vi "Begin.vi"(8 "error in":errorcluster) -> (0 "error out":errorcluster)   [LabVIEW 2014]
doc: "Called before other user functions, this VI is expected to open initial I/O refnums, load in file data, and do all program initialization. Notice that the <B>error out</B> terminal is simply used for data flow. Wiring it to other structures or subVIs ensures that this VI runs first."
uses:
  <vilib>/Rock Robotics/WPI/SafetyOutput/WPI_SafetyOutputConfigMenu.ctl
  <vilib>/Rock Robotics/WPI/DriverStation/WPI_DriverStationRobotMode2.ctl
  <vilib>/Rock Robotics/SystemInterfaces/AI/FPGA_AIGyroChannel.ctl
  <vilib>/Rock Robotics/SystemInterfaces/AI/FPGA_AIChannel.ctl
  Utilities/Sensor Refname.ctl
  <vilib>/Rock Robotics/SystemInterfaces/DIO/FPGA_DIOChannel.ctl
  Utilities/Refname.ctl
  <vilib>/Rock Robotics/WPI/Joystick/WPI_JoystickDeviceEnum.ctl
  <vilib>/Rock Robotics/WPI/CAN/TalonSRX/WPI_CANTalonSRX_APIControlMode.ctl
  <vilib>/Rock Robotics/WPI/CAN/TalonSRX/WPI_CANTalonSRX_APIFeedbackSelect.ctl
  Robot Global Data.vi
  <vilib>/Rock Robotics/WPI/RobotDrive/WPI_RobotDriveOpen4MotorWithCANTalonSRX.vi
  <vilib>/Rock Robotics/Network Tables/SD Write String.vi
  <vilib>/Rock Robotics/WPI/Switch/WPI_SwitchOpenLimit.vi
  Utilities/Sensor Refname to String.vi
  Utilities/RefnameToString.vi
  <vilib>/Rock Robotics/WPI/Ultrasonic/WPI_SonarMB1010AnalogOpen.vi
  <vilib>/Rock Robotics/WPI/Ultrasonic/WPI_SonarMB1010AnalogRefNum Registry Set.vi
  <vilib>/Rock Robotics/WPI/MotorControl/WPI_MotorControlOpenCANTalonSRX.vi
  <vilib>/Rock Robotics/WPI/Accelerometer/InternalAccelerometer/WPI_AccelerometerInternalOpen.vi
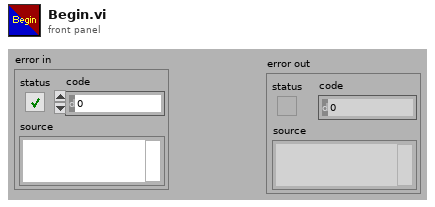
[diagram p1: front panel]
types:
  T1 = typedef "Refname.ctl" = enum16{"Gamepad 1", "Gamepad 2", "Drive Motors", "Strafe Motor", "Arm Clapper Motor", "Arm Angle", "Arm Belt Left", "Arm Belt Right", "Elevator 1", "Elevator 2", "Wiper"}
  T2 = cluster{"Refname":T1, "Device":u8, "Invert?":bool}[]
  T3 = typedef "WPI_JoystickDeviceEnum.ctl" = enum16{"USB 0", "USB 1", "USB 2", "USB 3", "USB 4", "USB 5"}
  T4 = typedef "Sensor Refname.ctl" = enum16{"Gyro", "Elevator Top LS", "Elevator Bottom LS", "Claw Outside LS", "Left Drive Encoder", "Right Drive Encoder", "Strafe Encoder", "Elevator Encoder", "Ultrasonic Forward", "Ultrasonic Back", "Arm Angle POT", "Arm Clapper POT", "Accelerometer", "Tote LS", "DIP 1", "DIP 2", "DIP 3", "DIP 4"}
  T5 = typedef "FPGA_AIChannel.ctl" = enum8{"AI 0", "AI 1", "AI 2", "AI 3", "AI MXP 0", "AI MXP 1", "AI MXP 2", "AI MXP 3", "Invalid"}
  T6 = cluster{"Sensor Refname":T4, "Analog Channel":T5}[]
  T7 = typedef "FPGA_DIOChannel.ctl" = enum8{"DIO 0", "DIO 1", "DIO 2", "DIO 3", "DIO 4", "DIO 5", "DIO 6", "DIO 7", "DIO 8", "DIO 9", "DIO MXP 0", "DIO MXP 1", "DIO MXP 2", "DIO MXP 3", "DIO MXP 4", "DIO MXP 5", "DIO MXP 6", "DIO MXP 7", "DIO MXP 8", "DIO MXP 9", "DIO MXP 10", "DIO MXP 11", "DIO MXP 12", "DIO MXP 13", "DIO MXP 14", "DIO MXP 15", "Invalid"}
  T8 = typedef "FPGA_AIGyroChannel.ctl" = enum8{"AI 0", "AI 1", "Invalid"}
  T9 = typedef "WPI_DriverStationRobotMode2.ctl" = enum16{"Autonomous Disabled", "Autonomous Enabled", "Teleop Disabled", "Teleop Enabled", "Disconnected", "Finish", "Test Disabled", "Test Enabled", "Emergency Stopped"}
  T10 = typedef "WPI_SafetyOutputConfigMenu.ctl" = enum16{"Enable", "Disable"}
  T11 = typedef "WPI_RobotDriveDevRef.ctl" = cluster{"DevStatus":errorcluster, "Motors[]":T12[], "Square Inputs":bool, "Max Output":dbl}
  T12 = typedef "WPI_MotorControlDeviceRef.ctl" = cluster{"DeviceStatus":errorcluster, "Type":T13, "PWM":cluster{"Controller":T14, "PWM Channel":T15, "DeadBand":T16}, "CAN":cluster{"Device Number":u8, "Control Mode":T17, "Semaphore":T18, "Max Vout":dbl, "TalonSRX Control Mode":T19}, "Invert":bool, "TransformRef":T20, "InvTransformRef":T20}
  T13 = typedef "WPI_MotorControlType.ctl" = enum16{"PWM", "CAN", "CANTalonSRX"}
  T14 = typedef "FPGA_TypedefDigitalModule.ctl" = enum16{"Controller 1"}
  T15 = typedef "FPGA_DIOPWMChannel.ctl" = enum8{"PWM 0", "PWM 1", "PWM 2", "PWM 3", "PWM 4", "PWM 5", "PWM 6", "PWM 7", "PWM 8", "PWM 9", "PWM MXP 0", "PWM MXP 1", "PWM MXP 2", "PWM MXP 3", "PWM MXP 4", "PWM MXP 5", "PWM MXP 6", "PWM MXP 7", "PWM MXP 8", "PWM MXP 9", "Invalid"}
  T16 = typedef "WPI_PWMDeadband.ctl" = cluster{"Name":string, "maxPositivePwm":i32, "minPositivePwm":i32, "centerPwm":i32, "maxNegativePwm":i32, "minNegativePwm":i32, "angularRange":u16}
  T17 = typedef "WPI_CANJaguar_ControlMode.ctl" = enum8{"Percent VBus", "Current", "Speed", "Position", "Voltage"}
  T18 = typedef "Semaphore RefNum" = refnum<k1>
  T19 = typedef "WPI_CANTalonSRX_APIControlMode.ctl" = enum8{"Percent VBus", "Speed", "Position", "Slave", "Unchanged / Invalid"}
  T20 = typedef "WPI_PWMTransform_ConPane.ctl" = refnum<vi>
  T21 = typedef "WPI_CANTalonSRX_APIFeedbackSelect.ctl" = enum16{"Digital Quadrature Encoder", "Analog Potentiometer", "Analog Encoder"}
  T22 = typedef "WPI_AccelerometerDevRef.ctl" = cluster{"DevStatus":errorcluster, "Controller":T23, "Scaling":T24, "Analog Channels":T25, "I2C Bus":T26, "SPI Bus":T27, "Accel Range":T28, "ADXL345 Axes":T29, "Handle":i32, "Device Address":u8, "Accel Type":enum16{"Analog", "ADXL345 I2C", "ADXL345 SPI", "Internal"}}
  T23 = typedef "FPGA_TypedefAnalogModule.ctl" = enum16{"Controller 1"}
  T24 = typedef "WPI_AccelerometerScaling.ctl" = cluster{"Gain (VoltsPerG)":dbl, "Center Voltage":dbl}
  T25 = typedef "WPI_AccelerometerAnalogChannels.ctl" = cluster{"X-Axis":T5, "Y-Axis":T5, "Z-Axis":T5}
  T26 = typedef "i2c_bus.ctl" = enum16{"I2C On-Board", "I2C MXP", "Invalid"}
  T27 = typedef "spi_bus.ctl" = enum16{"SPI On-Board, CS0", "SPI On-Board, CS1", "SPI On-Board, CS2", "SPI On-Board, CS3", "SPI MXP", "Invalid"}
  T28 = typedef "ADXL345 Range.ctl" = u8
  T29 = typedef "WPI_AccelerometerADXL345 Axes.ctl" = cluster{"X-Axis":bool, "Y-Axis":bool, "Z-Axis":bool}
  T30 = typedef "WPI_SonarMB1010AnalogDeviceRef.ctl" = cluster{"AIDeviceRef":T31, "Scaling factor (V/in)":dbl, "Average Bits":u8}
  T31 = typedef "WPI_AnalogChannelDevRef.ctl" = cluster{"DevStatus":errorcluster, "Controller":T23, "Analog Channel":T5}
  T32 = typedef "WPI_SwitchDevRef.ctl" = cluster{"DevStatus":errorcluster, "DIO Channel":T7, "Controller":T14, "CntIndex":T33, "Normally Closed":bool}
  T33 = typedef "FPGA_CounterCtrSystemIndex.ctl" = enum8{"Ctr 0", "Ctr 1", "Ctr 2", "Ctr 3", "Ctr 4", "Ctr 5", "Ctr 6", "Ctr 7", "Invalid"}
  T34 = typedef "WPI_JoystickDevRef.ctl" = cluster{"Device":T3}
  T35 = typedef "WPI_PotentiometerDevRef.ctl" = cluster{"DevStatus":errorcluster, "Controller":T23, "Analog Channel":T5, "Invert Output":bool}
  T36 = typedef "WPI_GyroDevRef.ctl" = cluster{"DevStatus":errorcluster, "Analog Module":T23, "Analog Channel":T5, "Offset":dbl, "Gain (VoltsPerDegree/Second)":dbl}
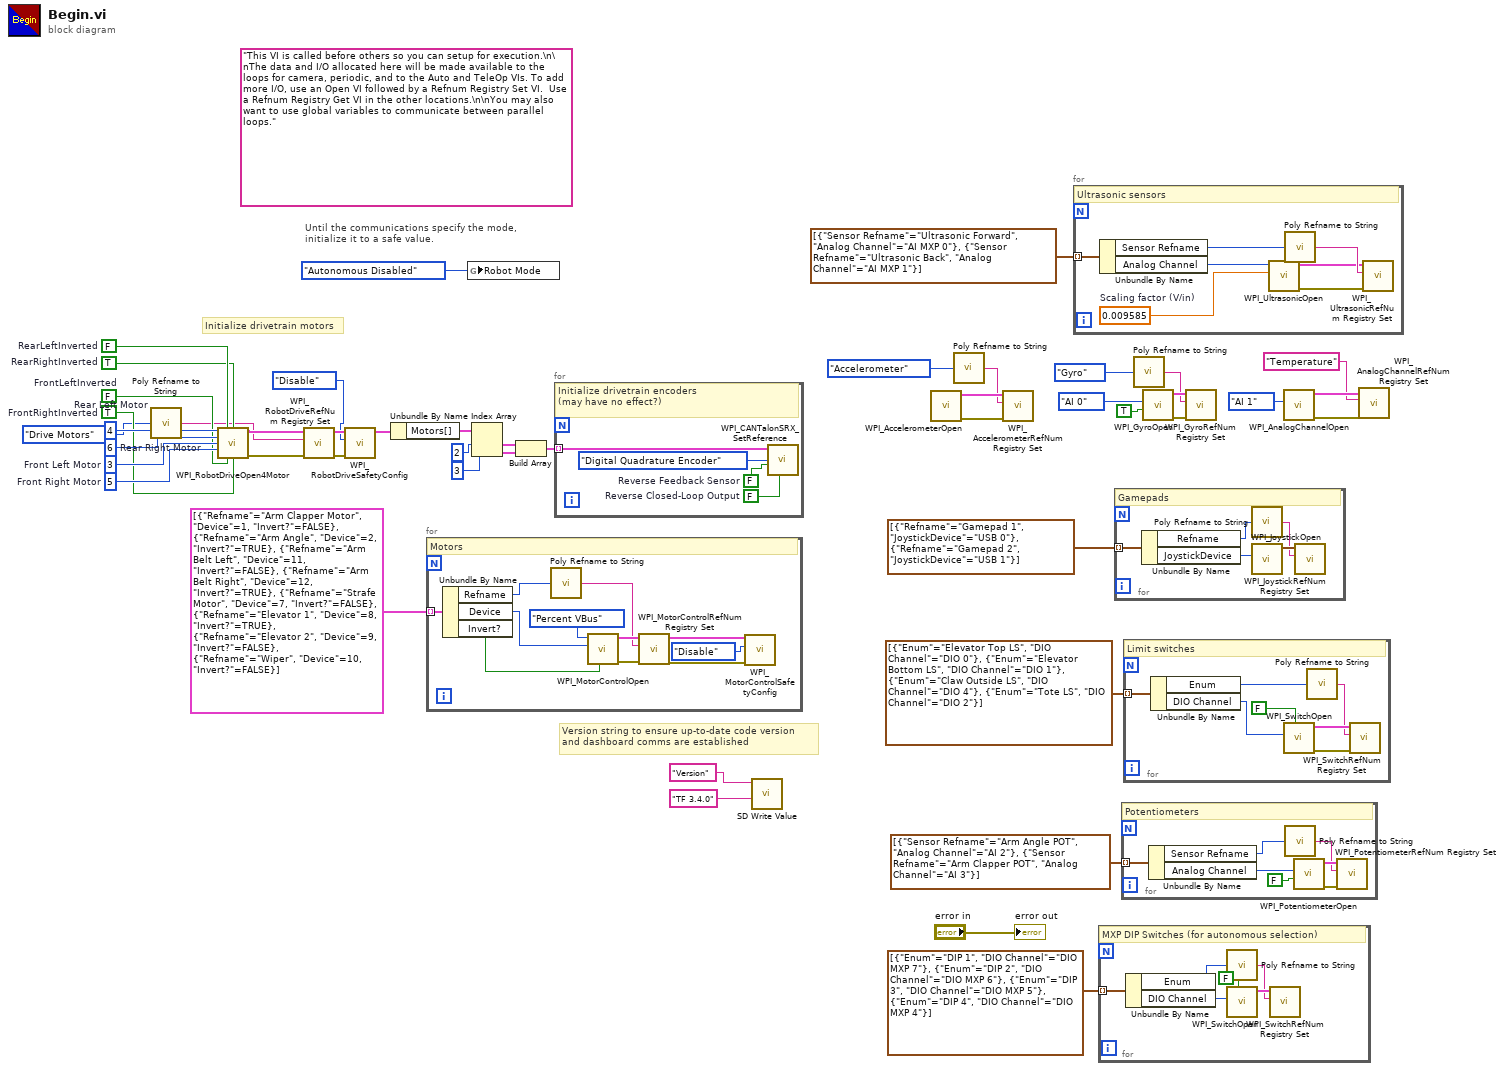
[diagram p0: block diagram]
diagram:
  w32 = TRUE  # RearRightInverted
  w33 = FALSE  # FrontLeftInverted
  w34 = TRUE  # FrontRightInverted
  w35 = FALSE  # RearLeftInverted
  w37 = u8 5  # Front Right Motor
  w38 = u8 3  # Front Left Motor
  w39 = u8 6  # Rear Right Motor
  w40 = u8 4  # Rear Left Motor
  (unwired) "This VI is called before others so you can setup for execution.\n\nThe data and I/O allocated here will be made available to the loops for camera, periodic, and to the Auto and TeleOp VIs. To add more I/O, use an Open VI followed by a Refnum Registry Set VI.  Use a Refnum Registry Get VI in the other locations.\n\nYou may also want to use global variables to communicate between parallel loops."
  # "Version string to ensure up-to-date code version\nand dashboard comms are established"
  # "Initialize drivetrain motors"
  # "Until the communications specify the mode,\ninitialize it to a safe value."
  n1 = call-poly "Poly Refname to String.vi"("Enum"=Refname."Drive Motors" ("Refname")) -> ("Refname"=w19:string)
  n2 = call-poly <vilib>:"WPI_RobotDriveOpen4Motor.vi"("Rear Left Motor"=w40, "Rear Left Motor Inverted"=w35, "Rear Right Motor Inverted"=w32, "Rear Right Motor"=w39, "Front Left Motor"=w38, "Front Right Motor"=w37, "Front Left Motor Inverted"=w33, "Front Right Motor Inverted"=w34) -> ("RobotDriveDevRef"=w46:T11, "error out"=w45:errorcluster)  [unwired: 6 in]
  n3 = call <vilib>:"WPI_RobotDriveRefNum Registry Set.vi"("error in (no error)"=w45, "refnum name"=w19, "RobotDriveDevRef"=w46) -> ("error out"=w36:errorcluster, "RobotDriveDevRef"=w44:T11)  [unwired: 7 out]
  n4 = call <vilib>:"WPI_RobotDriveSafetyConfig.vi"("error in (no error)"=w36, "mode"=WPI_SafetyOutputConfigMenu."Disable", "RobotDriveDevRef"=w44) -> ("RobotDriveDevRef"=w26:T11)  [unwired: 7 in, 1 out]
  n5 = Unbundle By Name(w26) -> ("Motors[]"=w25:T12[])
  n6 = for {
    tunnel: T2 [{"Refname"=enum."Arm Clapper Motor", "Device"=1, "Invert?"=FALSE}, {"Refname"=enum."Arm Angle", "Device"=2, "Invert?"=TRUE}, {"Refname"=enum."Arm Belt Left", "Device"=11, "Invert?"=FALSE}, {"Refname"=enum."Arm Belt Right", "Device"=12, "Invert?"=TRUE}, {"Refname"=enum."Strafe Motor", "Device"=7, "Invert?"=FALSE}, {"Refname"=enum."Elevator 1", "Device"=8, "Invert?"=TRUE}, {"Refname"=enum."Elevator 2", "Device"=9, "Invert?"=FALSE}, {"Refname"=enum."Wiper", "Device"=10, "Invert?"=FALSE}] -> [w47] mode=indexing
    # "Motors"
    n7 = Unbundle By Name(w47) -> ("Refname"=w50:T1, "Device"=w49:u8, "Invert?"=w48:bool)
    n8 = call-poly "Poly Refname to String.vi"("Enum"=w50) -> ("Refname"=w51:string)
    n9 = call-poly <vilib>:"WPI_MotorControlOpen.vi"("Invert"=w48, "Device Number"=w49, "Control Mode"=WPI_CANTalonSRX_APIControlMode."Percent VBus") -> ("error out"=w57:errorcluster, "MotorControlDeviceRef"=w55:T12)  [unwired: 7 in]
    n10 = call <vilib>:"WPI_MotorControlRefNum Registry Set.vi"("error in (no error)"=w57, "refnum name"=w51, "MotorControlDevRef"=w55) -> ("error out"=w53:errorcluster, "MotorControlDevRef"=w54:T12)  [unwired: 7 in]
    n11 = call <vilib>:"WPI_MotorControlSafetyConfig.vi"("error in (no error)"=w53, "mode"=WPI_SafetyOutputConfigMenu."Disable", "MotorControlDevRef"=w54) -> ()  [unwired: 7 in, 2 out]
  }
  n12 = global write "Robot Global Data.vi" "Robot Mode"(WPI_DriverStationRobotMode2."Autonomous Disabled" ("Robot Mode")) -> ()
  n13 = Index Array(array=w25, index #1=2 ("index"), index #2=3 ("index")) -> (element #1=w22:T12, element #2=w21:T12)
  n14 = Build Array(w22, w21) -> (w20:T12[])
  n15 = for {
    tunnel: w20 -> [w60] mode=indexing
    w58 = FALSE  # Reverse Closed-Loop Output
    w59 = FALSE  # Reverse Feedback Sensor
    # "Initialize drivetrain encoders\n(may have no effect?)"
    n16 = call <vilib>:"WPI_CANTalonSRX_SetReference.vi"("Reverse Closed-Loop Output"=w58, "Reverse Feedback Sensor"=w59, "Feedback Reference"=WPI_CANTalonSRX_APIFeedbackSelect."Digital Quadrature Encoder", "CAN Talon SRX Ref"=w60) -> ()  [unwired: 6 in, 2 out]
  }
  n17 = call-poly <vilib>:"SD Write Value.vi"("String"="TF 3.4.0", "Name"="Version") -> ()  [unwired: 8 in, 2 out]
  n18 = call-poly <vilib>:"WPI_AccelerometerOpen.vi"() -> ("error out"=w18:errorcluster, "AccelerometerDevRef"=w17:T22)  [unwired: 10 in]
  n19 = call-poly "Poly Refname to String.vi"("Sensor Refnames"=Sensor_Refname."Accelerometer" ("Sensor Refname")) -> ("Refname"=w16:string)
  n20 = call <vilib>:"WPI_AccelerometerRefNum Registry Set.vi"("error in (no error)"=w18, "refnum name"=w16, "AccelerometerDevRef"=w17) -> ()  [unwired: 7 in, 2 out]
  n21 = for {
    tunnel: T6 [{"Sensor Refname"=enum."Ultrasonic Forward", "Analog Channel"=enum."AI MXP 0"}, {"Sensor Refname"=enum."Ultrasonic Back", "Analog Channel"=enum."AI MXP 1"}] -> [w66] mode=indexing
    w65 = 0.009585  # Scaling factor (V/in)
    # "Ultrasonic sensors"
    n22 = Unbundle By Name(w66) -> ("Sensor Refname"=w67:T4, "Analog Channel"=w62:T5)
    n23 = call-poly <vilib>:"WPI_UltrasonicOpen.vi"("Scaling factor (V/in)"=w65, "Analog Channel"=w62) -> ("error out"=w64:errorcluster, "SonarMB1010AnalogDevRef"=w63:T30)  [unwired: 8 in]
    n24 = call-poly "Poly Refname to String.vi"("Sensor Refnames"=w67) -> ("Refname"=w68:string)
    n25 = call-poly <vilib>:"WPI_UltrasonicRefNum Registry Set.vi"("error in (no error)"=w64, "refnum name"=w68, "SonarMB1010AnalogDevRef"=w63) -> ()  [unwired: 7 in, 2 out]
  }
  n26 = for {
    tunnel: cluster{"Enum":T4, "DIO Channel":T7}[] [{"Enum"=enum."DIP 1", "DIO Channel"=enum."DIO MXP 7"}, {"Enum"=enum."DIP 2", "DIO Channel"=enum."DIO MXP 6"}, {"Enum"=enum."DIP 3", "DIO Channel"=enum."DIO MXP 5"}, {"Enum"=enum."DIP 4", "DIO Channel"=enum."DIO MXP 4"}] -> [w74] mode=indexing
    # "MXP DIP Switches (for autonomous selection)"
    n27 = Unbundle By Name(w74) -> ("Enum"=w73:T4, "DIO Channel"=w72:T7)
    n28 = call-poly "Poly Refname to String.vi"("Sensor Refnames"=w73) -> ("Refname"=w70:string)
    n29 = call-poly <vilib>:"WPI_SwitchOpen.vi"("Normally Closed"=FALSE, "DIO Channel"=w72) -> ("SwitchDevRef"=w71:T32)  [unwired: 8 in, 1 out]
    n30 = call <vilib>:"WPI_SwitchRefNum Registry Set.vi"("refnum name"=w70, "SwitchDevRef"=w71) -> ()  [unwired: 8 in, 2 out]
  }
  n31 = for {
    tunnel: cluster{"Refname":T1, "JoystickDevice":T3}[] [{"Refname"=enum."Gamepad 1", "JoystickDevice"=enum."USB 0"}, {"Refname"=enum."Gamepad 2", "JoystickDevice"=enum."USB 1"}] -> [w75] mode=indexing
    # "Gamepads"
    n32 = Unbundle By Name(w75) -> ("Refname"=w77:T1, "JoystickDevice"=w76:T3)
    n33 = call-poly "Poly Refname to String.vi"("Enum"=w77) -> ("Refname"=w78:string)
    n34 = call <vilib>:"WPI_JoystickOpen.vi"("JoystickDevice"=w76) -> ("JoystickDevRef"=w79:T34)  [unwired: 10 in]
    n35 = call <vilib>:"WPI_JoystickRefNum Registry Set.vi"("refnum name"=w78, "JoystickDevRef"=w79) -> ()  [unwired: 8 in, 2 out]
  }
  n36 = for {
    tunnel: T6 [{"Sensor Refname"=enum."Arm Angle POT", "Analog Channel"=enum."AI 2"}, {"Sensor Refname"=enum."Arm Clapper POT", "Analog Channel"=enum."AI 3"}] -> [w80] mode=indexing
    # "Potentiometers"
    n37 = Unbundle By Name(w80) -> ("Sensor Refname"=w82:T4, "Analog Channel"=w81:T5)
    n38 = call-poly "Poly Refname to String.vi"("Sensor Refnames"=w82) -> ("Refname"=w83:string)
    n39 = call <vilib>:"WPI_PotentiometerOpen.vi"("Invert Output"=FALSE, "Analog Channel"=w81) -> ("error out"=w84:errorcluster, "PotDevRef"=w86:T35)  [unwired: 8 in]
    n40 = call <vilib>:"WPI_PotentiometerRefNum Registry Set.vi"("error in (no error)"=w84, "refnum name"=w83, "PotDevRef"=w86) -> ()  [unwired: 7 in, 2 out]
  }
  n41 = for {
    tunnel: cluster{"Enum":T4, "DIO Channel":T7}[] [{"Enum"=enum."Elevator Top LS", "DIO Channel"=enum."DIO 0"}, {"Enum"=enum."Elevator Bottom LS", "DIO Channel"=enum."DIO 1"}, {"Enum"=enum."Claw Outside LS", "DIO Channel"=enum."DIO 4"}, {"Enum"=enum."Tote LS", "DIO Channel"=enum."DIO 2"}] -> [w87] mode=indexing
    # "Limit switches"
    n42 = Unbundle By Name(w87) -> ("Enum"=w89:T4, "DIO Channel"=w88:T7)
    n43 = call-poly <vilib>:"WPI_SwitchOpen.vi"("Normally Closed"=FALSE, "DIO Channel"=w88) -> ("error out"=w92:errorcluster, "SwitchDevRef"=w93:T32)  [unwired: 8 in]
    n44 = call-poly "Poly Refname to String.vi"("Sensor Refnames"=w89) -> ("Refname"=w91:string)
    n45 = call <vilib>:"WPI_SwitchRefNum Registry Set.vi"("error in (no error)"=w92, "refnum name"=w91, "SwitchDevRef"=w93) -> ()  [unwired: 7 in, 2 out]
  }
  n46 = call-poly "Poly Refname to String.vi"("Sensor Refnames"=Sensor_Refname."Gyro" ("Sensor Refname")) -> ("Refname"=w27:string)
  n47 = call <vilib>:"WPI_GyroOpen.vi"("Calibrate On Open"=TRUE, "Analog Channel"=FPGA_AIGyroChannel."AI 0") -> ("error out"=w29:errorcluster, "GyroDevRef"=w28:T36)  [unwired: 7 in, 1 out]
  n48 = call <vilib>:"WPI_GyroRefNum Registry Set.vi"("error in (no error)"=w29, "refnum name"=w27, "GyroDevRef"=w28) -> ()  [unwired: 7 in, 2 out]
  n49 = call <vilib>:"WPI_AnalogChannelOpen.vi"("Analog Channel"=FPGA_AIChannel."AI 1") -> ("error out"=w13:errorcluster, "AIDeviceRef"=w12:T31)  [unwired: 9 in]
  n50 = call <vilib>:"WPI_AnalogChannelRefNum Registry Set.vi"("error in (no error)"=w13, "refnum name"="Temperature", "AIDeviceRef"=w12) -> ()  [unwired: 7 in, 2 out]
  "error out" <- "error in"
